vi "TPNT_GetDev2Str.vi"(8 "error in (no error)":errorcluster, 11 "Object Refnum In":T1) -> (0 "error out":errorcluster, 2 "str out":string)   [LabVIEW 2016]
uses:
  TPNT_Refnum.ctl
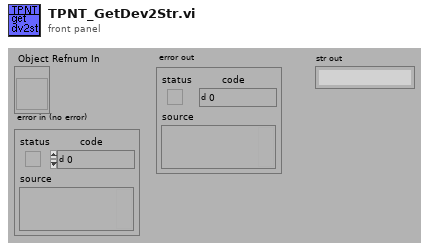
[diagram p1: front panel]
types:
  T1 = typedef "TPNT_Refnum.ctl" = refnum<vi>
  T2 = typedef "TPNT_DeviceTPs.ctl" = cluster{"device":string, "devupdate":dbl, "next_update":u32, "devinterface":string, "TPs":T3[], "Alarms":bool, "monitor":bool, "log sep":string}
  T3 = typedef "TPNT_TP.ctl" = cluster{"name":string, "type":string, "algor":string[], "update_rate":sgl, "Limits":T4, "Samples":T5, "next_update":u32, "Status":string, "monitor":bool, "error":bool, "Log":T6, "permissions":string, "ID":string}
  T4 = typedef "TPNT_Limits.ctl" = cluster{"Alarm Type":string, "Lower ":dbl, "Upper":dbl, "Nominal":dbl, "outrange":bool, "Check":bool, "latch":bool, "level":string}
  T5 = typedef "TPNT_Samples.ctl" = cluster{"samples":i32, "counter":i32, "Values":dbl[], "Current Value":string, "filter":string, "precision":u8}
  T6 = typedef "TPNT_Log.ctl" = cluster{"log":bool, "file":path, "type":string, "format":string, "updaterate":dbl, "nex_update":u32, "mode":string}
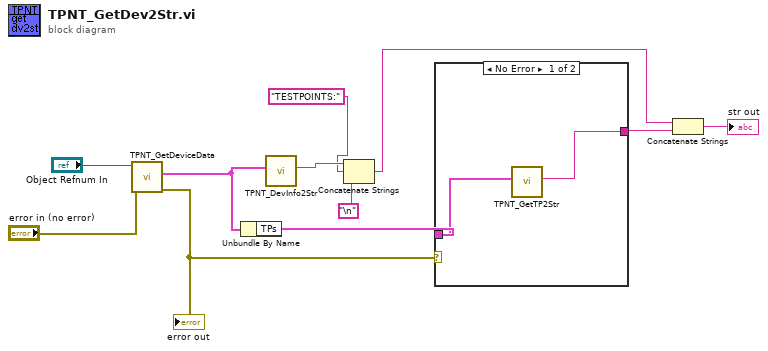
[diagram p0: block diagram]
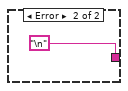
[diagram p2: hidden frame]
diagram:
  n1 = call "TPNT_GetDeviceData.vi"("error in (no error)"="error in (no error)", "Object Refnum In"="Object Refnum In") -> ("error out"=w4:errorcluster, "Object Data Out"=w11:T2)  [unwired: 8 out]
  "error out" <- w4
  n2 = Unbundle By Name(w11) -> ("TPs"=w5:T3[])
  n3 = call "TPNT_DevInfo2Str.vi"("Device In"=w11) -> ("TP out"=w7:string)  [unwired: 10 out]
  n4 = Concatenate Strings(w7, "TESTPOINTS:" ("string"), "\n") -> (w3:string)
  n5 = case shown="No Error" w4 {
    tunnel: w5 -> [w13 _]
    tunnel: [w12 "\n"] -> w2
    frame No Error {
      n6 = call "TPNT_GetTP2Str.vi"("TPs"=w13) -> ("String"=w12:string)  [unwired: 1 in, 9 out]
    }
    frame Error {
    }
  }
  n7 = Concatenate Strings(w3, w2) -> (→"str out":string)
